vi "First Step.vi"(8 "error in (no error)":errorcluster, 11 "Wavelength iHR320.lvclass in":refnum<class "Wavelength iHR320.lvclass">) -> (0 "error out":errorcluster, 2 "Current Position":dbl, 3 "Wavelength iHR320.lvclass out":refnum<class "Wavelength iHR320.lvclass">)   [LabVIEW 2009, in "Wavelength iHR320.lvclass"]
doc: "(Dynamic) Reset the instrument and prepare to scan. Go to step #0 - the first step. If desired, the scanner may do this in a different way than usual (i.e. by preparing to move a long distance, or reset to home position.)"
uses:
  Wavelength iHR320.lvclass
  Instruments/Spectrometer iHR320/Spectrometer iHR320.lvclass
  Scanner/Scanner.lvclass
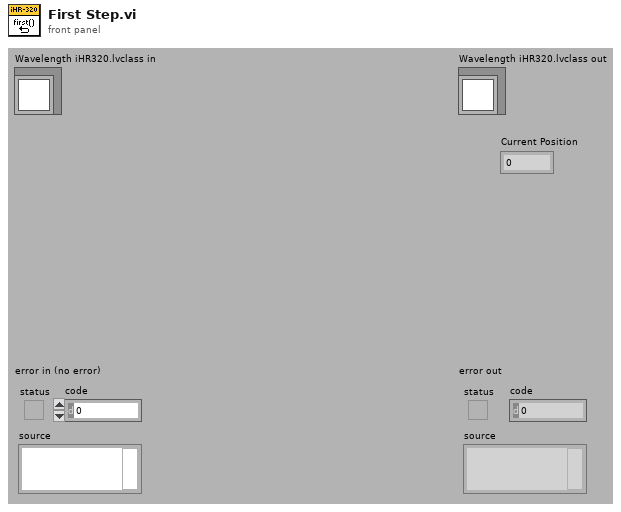
[diagram p1: front panel]
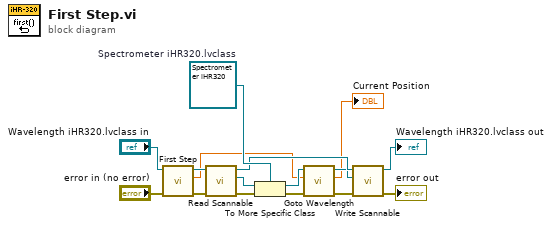
[diagram p0: block diagram]
diagram:
  w12 = refnum<class "Spectrometer iHR320.lvclass"> refnum  # Spectrometer iHR320.lvclass
  n1 = call-parent "First Step.vi"("error in (no error)"="error in (no error)", "Scanner.lvclass in"="Wavelength iHR320.lvclass in") -> ("error out"=w14:errorcluster, "Current Position"=w5:dbl, "Scanner.lvclass out"=w13:refnum<class "Wavelength iHR320.lvclass">)  [unwired: 7 in]
  n2 = call-dynamic "Read Scannable.vi"("error in (no error)"=w14, "Scanner.lvclass in"=w13) -> ("error out"=w11:errorcluster, "Scannable.lvclass"=w7:refnum<class "Scannable.lvclass">, "Scanner.lvclass out"=w10:refnum<class "Wavelength iHR320.lvclass">)  [unwired: 7 in]
  n3 = To More Specific Class(target class=w12, reference=w7, error in=w11) -> (specific class reference=w6:refnum<class "Spectrometer iHR320.lvclass">, error out=w4:errorcluster)
  n4 = call "Goto Wavelength.vi"("error in (no error)"=w4, "Target WL"=w5, "Spectrometer iHR320.lvclass In"=w6) -> ("error out"=w1:errorcluster, "Actual WL"=→"Current Position":dbl, "Spectrometer iHR320.lvclass Out"=w3:refnum<class "Spectrometer iHR320.lvclass">)  [unwired: 6 in]
  n5 = call-dynamic "Write Scannable.vi"("error in (no error)"=w1, "Scannable.lvclass"=w3, "Scanner.lvclass in"=w10) -> ("error out"=→"error out":errorcluster, "Scanner.lvclass out"=→"Wavelength iHR320.lvclass out":refnum<class "Wavelength iHR320.lvclass">)  [unwired: 7 in]
